vi "GetChannelSet.vi"(11 "Msg Data":string) -> (1 "ControlPara":dbl[][](array[numeric]), 3 "ChannelSetArray":T1[](array[typedef]) {"Enable" items=["不使能", "使能"]; "Wave" items=["0指令", "正弦波", "方波", "三角波", "常值", "波形数据", "白噪声", "正弦扫频", "梯度加载", "VMIC"]; "ChannelType" items=["标准波形跟踪"=1, "扫频测试"=2, "消除多余力"=3, "梯度加载"=4, "载荷谱跟踪"=5, "模拟输入跟踪"=9]; "ChannelStatus" items=["通道关", "位置通道", "加载通道"]})   [LabVIEW 2014]
uses:
  ChannelCommand.ctl
  Control 1.ctl
  WaveType.ctl
  MoterEnable.ctl
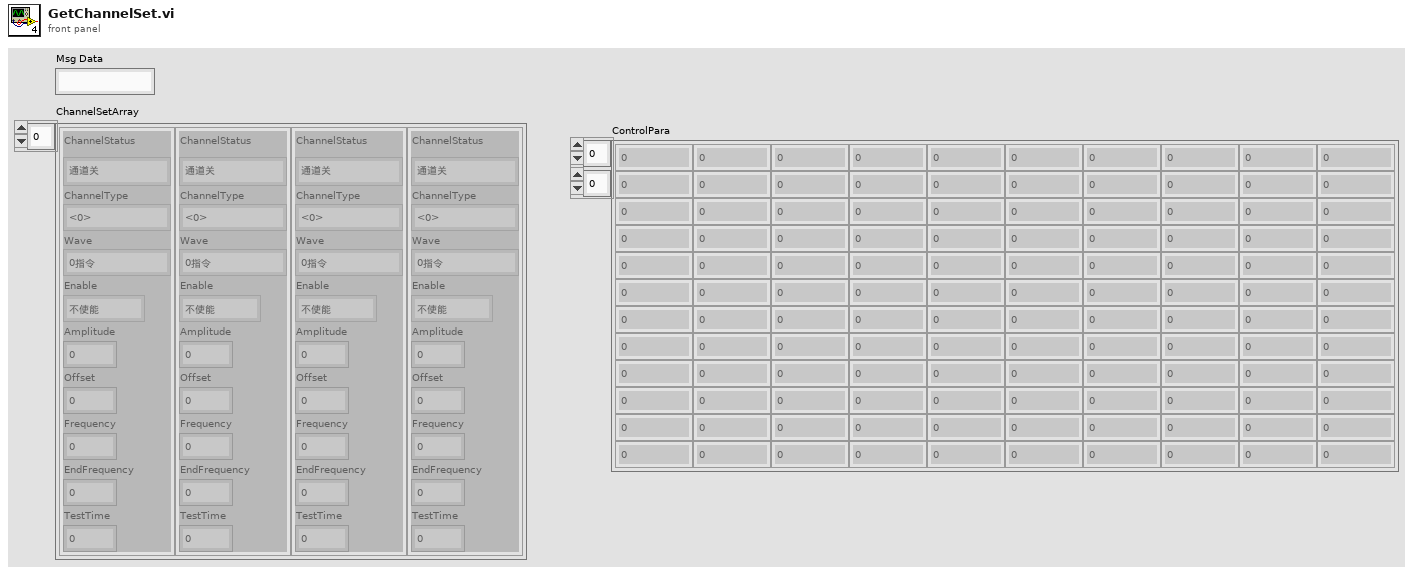
[diagram p1: front panel]
types:
  T1 = typedef "ChannelCommand.ctl" = cluster{"ChannelStatus":T2, "ChannelType":i32, "Wave":T3, "Enable":T4, "Amplitude":dbl, "Offset":dbl, "Frequency":dbl, "EndFrequency":dbl, "TestTime":dbl}
  T2 = typedef "Control 1.ctl" = i32
  T3 = typedef "WaveType.ctl" = i32
  T4 = typedef "MoterEnable.ctl" = u16
  T5 = enum16{"big-endian, network order", "native, host order", "little-endian"}
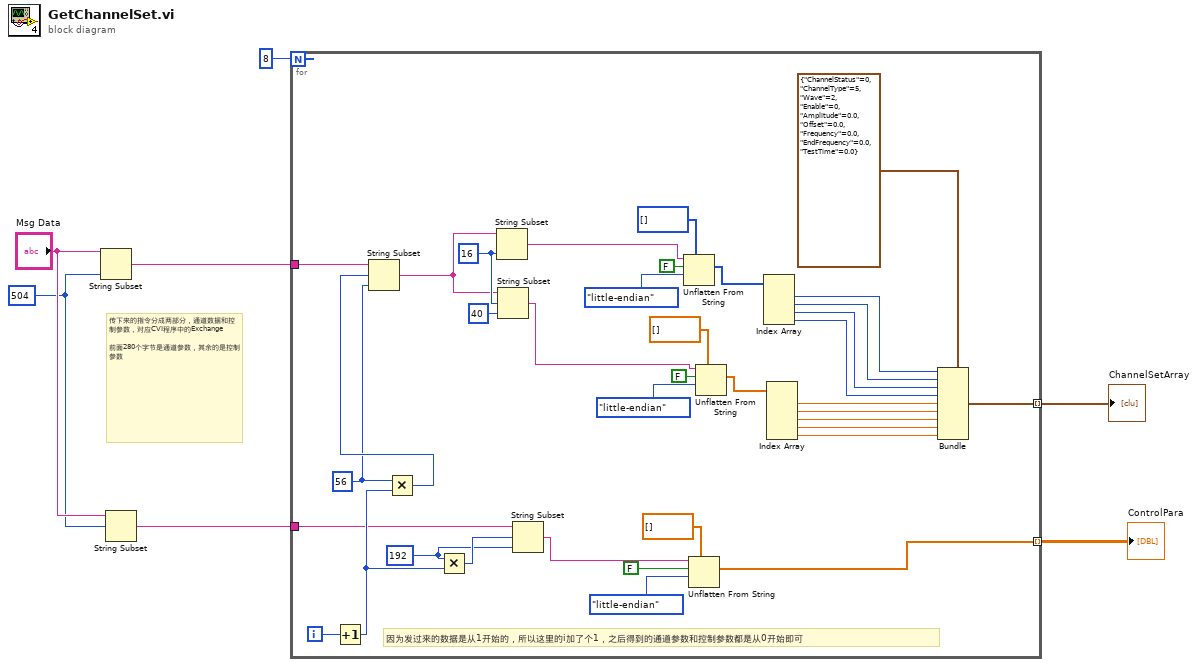
[diagram p0: block diagram]
diagram:
  w3 = 504 ("length (rest)")
  # "传下来的指令分成两部分，通道数据和控制参数，对应CVI程序中的Exchange\n\n前面280个字节是通道参数，其余的是控制参数"
  n1 = String Subset(string="Msg Data", length (rest)=w3) -> (substring=w5:string)  [unwired: 1 in]
  n2 = String Subset(string="Msg Data", offset (0)=w3) -> (substring=w2:string)  [unwired: 1 in]
  n3 = for {
    N: 8 -> [_]
    tunnel: [w44] -> w6 mode=indexing
    tunnel: w5 -> [w18]
    tunnel: w2 -> [w14]
    tunnel: [w9] -> w1 mode=indexing
    i -> [w37]
    w15 = 192 ("x")
    w35 = 56 ("x")
    w40 = 16 ("length (rest)")
    # "因为发过来的数据是从1开始的，所以这里的i加了个1，之后得到的通道参数和控制参数都是从0开始即可"
    n4 = Increment(x=w37) -> (x+1=w17:i32)
    n5 = Multiply(x=w35, y=w17) -> (x*y=w36:i32)
    n6 = String Subset(string=w18, offset (0)=w36, length (rest)=w35) -> (substring=w19:string)
    n7 = Multiply(x=w15, y=w17) -> (x*y=w16:i32)
    n8 = String Subset(string=w19, length (rest)=w40) -> (substring=w38:string)  [unwired: 1 in]
    n9 = String Subset(string=w19, offset (0)=w40, length (rest)=40 ("length (rest)")) -> (substring=w31:string)
    n10 = String Subset(string=w14, offset (0)=w16, length (rest)=w15) -> (substring=w10:string)
    n11 = Unflatten From String(type=i32[] [], binary string=w38, data includes array or string size? (T)=FALSE, byte order (0:big-endian, network order)=T5."little-endian") -> (value=w30:i32[])  [unwired: 1 in, 2 out]
    n12 = Unflatten From String(type=dbl[] [], binary string=w10, data includes array or string size? (T)=FALSE, byte order (0:big-endian, network order)=T5."little-endian") -> (value=w9:dbl[])  [unwired: 1 in, 2 out]
    n13 = Unflatten From String(type=dbl[] [], binary string=w31, data includes array or string size? (T)=FALSE, byte order (0:big-endian, network order)=T5."little-endian") -> (value=w25:dbl[])  [unwired: 1 in, 2 out]
    n14 = Index Array(array=w30) -> (element #1=w29:i32, element #2=w28:i32, element #3=w27:i32, element #4=w26:i32)  [unwired: 4 in]
    n15 = Index Array(array=w25) -> (element #1=w24:dbl, element #2=w23:dbl, element #3=w22:dbl, element #4=w21:dbl, element #5=w20:dbl)  [unwired: 5 in]
    n16 = Bundle(cluster=T1 {"ChannelStatus"=0, "ChannelType"=5, "Wave"=2, "Enable"=0, "Amplitude"=0.0, "Offset"=0.0, "Frequency"=0.0, "EndFrequency"=0.0, "TestTime"=0.0} ("Cluster"), "ChannelStatus"=w29, "ChannelType"=w28, "Wave"=w27, "Enable"=w26, "Amplitude"=w24, "Offset"=w23, "Frequency"=w22, "EndFrequency"=w21, "TestTime"=w20) -> (w44:T1)
  }
  "ChannelSetArray" <- w6
  "ControlPara" <- w1
